vi "ReceiveCalibrationData.vi"(6 "Timeout ms":i32=1, 7 "UDP Input":T1) -> (0 "Error Out":errorcluster, 1 "CalibrationData":cluster{"value":i8, "motor":i8}, 2 "Did Receive":bool, 3 "UDP Output":T1)   [LabVIEW 2019]
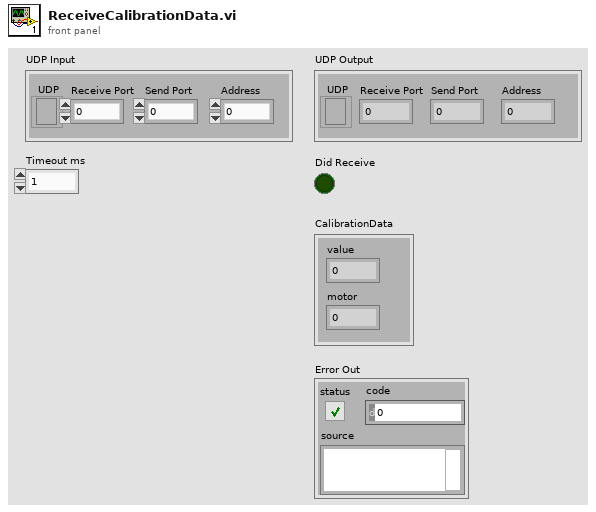
[diagram p1: front panel]
types:
  T1 = cluster{"UDP":refnum<k16>, "Receive Port":i32, "Send Port":i32, "Address":i64}
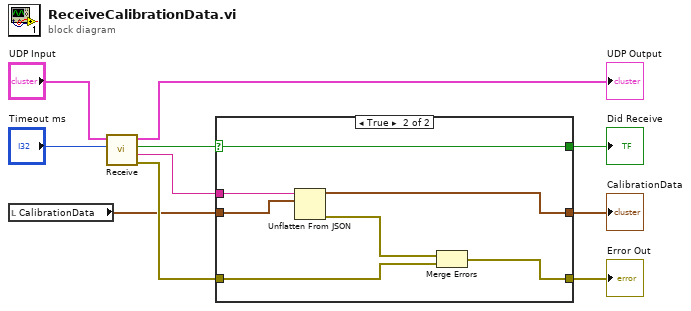
[diagram p0: block diagram]
diagram:
  n1 = local read "CalibrationData"() -> (w1:cluster{"value":i8, "motor":i8})
  n2 = call "Receive.vi"("Timeout ms"="Timeout ms", "UDP Input"="UDP Input") -> ("Error Out"=w3:errorcluster, "Received Data"=w7:string, "Did Receive"=w6:bool, "UDP Output"=→"UDP Output":T1)  [unwired: 2 in]
  n3 = case shown="True" w6 {
    selector: w6 -> [w13 w20]
    tunnel: w7 -> [_ w18]
    tunnel: [w13 w20] -> w5
    tunnel: [w12 w15] -> w4
    tunnel: w3 -> [w12 w16]
    tunnel: [w11 w14] -> w2
    tunnel: w1 -> [w11 w17]
    frame False {
    }
    frame True {
      n4 = Unflatten From JSON(JSON string=w18, type and defaults=w17) -> (value=w14:cluster{"value":i8, "motor":i8}, error out=w19:errorcluster)  [unwired: 5 in]
      n5 = Merge Errors(w19, w16) -> (w15:errorcluster)
    }
  }
  "Error Out" <- w4
  "Did Receive" <- w5
  "CalibrationData" <- w2
